vi "Test - Monitor Slip.vi"(8 "error in (no error)":errorcluster, 11 "Cluster":T1={"Preslip Sequence"=[], "Step No"=0, "Step Value"={"Sr.no"=0, "Log?"=FALSE, "Step"="", "Type"="", "Channel"="", "Value"=0.0, "Para1"=0.0, "Para2"=0.0, "Limit1"=0.0, "Limit2"=0.0, "Comparision Mode"="", "Timeout"=0.0}, "Slip Parameter"=[], "Slip Timer"=0.0, "Postslip Sequence"=[], "Postslip ?"=FALSE, "Step Result"={"Step Name"="", "Value"=0.0, "Success ?"=TRUE, "Stop Seq ?"=TRUE, "Abort"=TRUE, "Sr.No"=0}}) -> (0 "error out":errorcluster, 2 "Slip Occured ?":bool)   [LabVIEW 2017]
uses:
  Test - Message cluster.ctl
  Test - Step config.ctl
  Test - Step Result.ctl
  SubVIs/SubVI - Global.vi
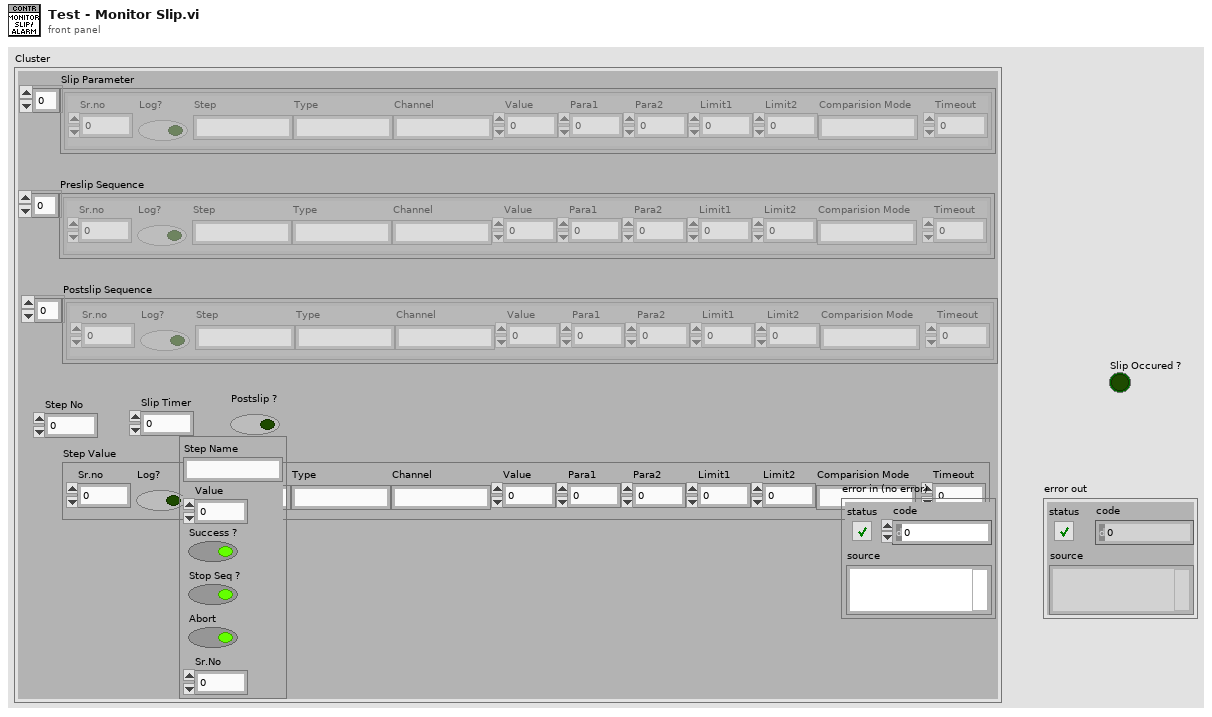
[diagram p1: front panel]
types:
  T1 = typedef "Test - Message cluster.ctl" = cluster{"Preslip Sequence":T2[], "Step No":i32, "Step Value":T2, "Slip Parameter":T2[], "Slip Timer":dbl, "Postslip Sequence":T2[], "Postslip ?":bool, "Step Result":T3}
  T2 = typedef "Test - Step config.ctl" = cluster{"Sr.no":i32, "Log?":bool, "Step":string, "Type":string, "Channel":string, "Value":dbl, "Para1":dbl, "Para2":dbl, "Limit1":dbl, "Limit2":dbl, "Comparision Mode":string, "Timeout":dbl}
  T3 = typedef "Test - Step Result.ctl" = cluster{"Step Name":string, "Value":dbl, "Success ?":bool, "Stop Seq ?":bool, "Abort":bool, "Sr.No":i32}
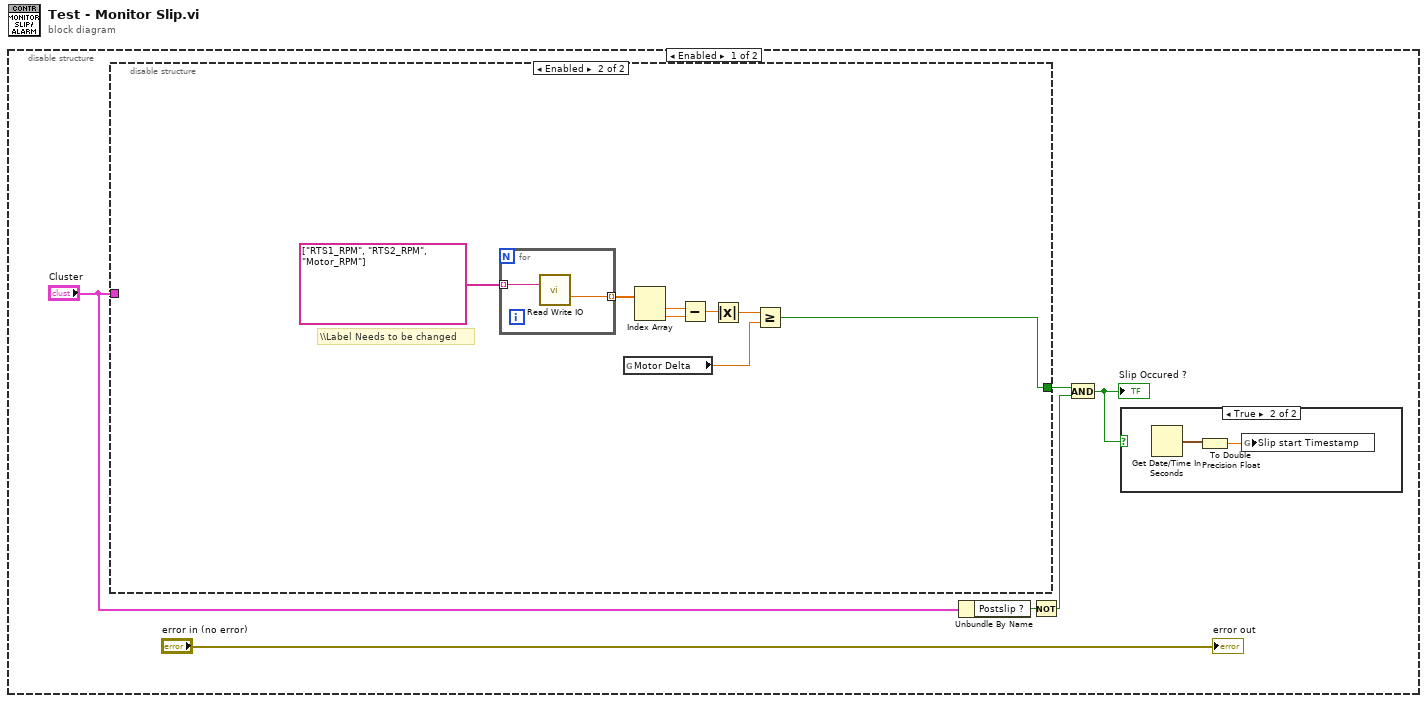
[diagram p0: block diagram]
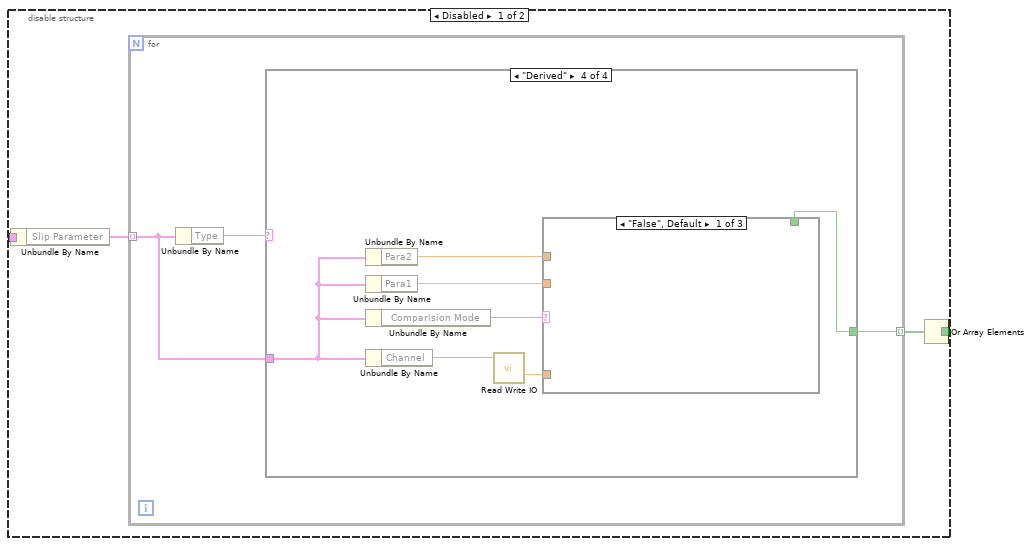
[diagram p2: hidden frame]
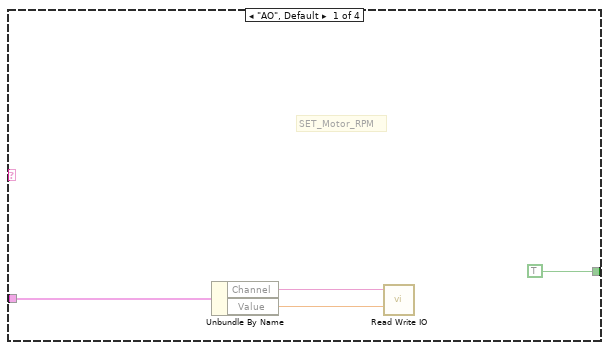
[diagram p3: hidden frame]
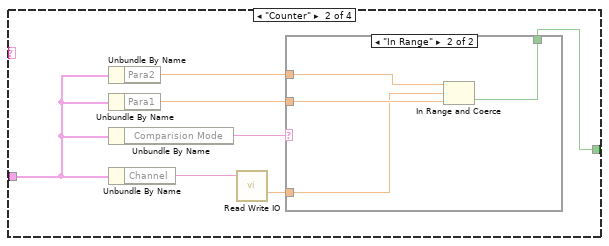
[diagram p4: hidden frame]
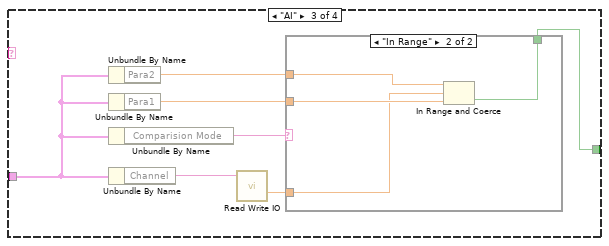
[diagram p6: hidden frame]
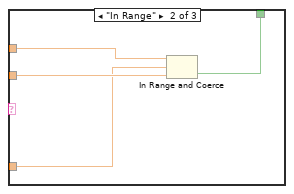
[diagram p8: hidden frame]
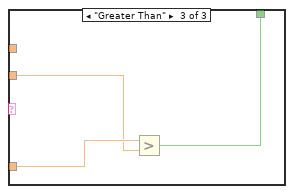
[diagram p9: hidden frame]
diagram:
  n1 = disable-structure shown="Enabled" {
    frame Enabled {
      n2 = disable-structure shown="Enabled" {
        disable-tunnel: "Cluster" -> [w8 _]
        disable-tunnel: [w7 w54] -> w2
        frame Disabled {
          n3 = Unbundle By Name(w8) -> ("Slip Parameter"=w9:T2[])
          n4 = for {
            tunnel: [w12] -> w10 mode=indexing
            tunnel: w9 -> [w11] mode=indexing
            n5 = Unbundle By Name(w11) -> ("Type"=w13:string)
            n6 = case shown="\"Derived\"" w13 {
              tunnel: w11 -> [w17 w24 w35 w46]
              tunnel: [TRUE w23 w34 w45] -> w12
              frame "AO", Default {
                # "SET_Motor_RPM"
                n7 = Unbundle By Name(w17) -> ("Channel"=w16:string, "Value"=w15:dbl)
                n8 = call "Read Write IO.vi"("Tag Name"=w16, "Value In"=w15) -> ()  [unwired: 11 in, 3 out]
              }
              frame "Counter" {
                n9 = Unbundle By Name(w24) -> ("Para2"=w19:dbl)
                n10 = Unbundle By Name(w24) -> ("Para1"=w18:dbl)
                n11 = Unbundle By Name(w24) -> ("Comparision Mode"=w21:string)
                n12 = Unbundle By Name(w24) -> ("Channel"=w22:string)
                n13 = call "Read Write IO.vi"("Tag Name"=w22) -> ("Value Out"=w20:dbl)  [unwired: 12 in, 2 out]
                n14 = case shown="\"In Range\"" w21 {
                  tunnel: w20 -> [_ w26]
                  tunnel: w19 -> [_ w28]
                  tunnel: w18 -> [_ w27]
                  tunnel: [_ w25] -> w23
                  frame "False", Default {
                  }
                  frame "In Range" {
                    n15 = In Range and Coerce(upper limit=w28, x=w26, lower limit=w27) -> (In Range?=w25:bool)  [unwired: 1 out]
                  }
                }
              }
              frame "AI" {
                n16 = Unbundle By Name(w35) -> ("Para2"=w30:dbl)
                n17 = Unbundle By Name(w35) -> ("Para1"=w29:dbl)
                n18 = Unbundle By Name(w35) -> ("Comparision Mode"=w32:string)
                n19 = Unbundle By Name(w35) -> ("Channel"=w33:string)
                n20 = call "Read Write IO.vi"("Tag Name"=w33) -> ("Value Out"=w31:dbl)  [unwired: 12 in, 2 out]
                n21 = case shown="\"In Range\"" w32 {
                  tunnel: w31 -> [_ w37]
                  tunnel: w30 -> [_ w39]
                  tunnel: w29 -> [_ w38]
                  tunnel: [_ w36] -> w34
                  frame "False", Default {
                  }
                  frame "In Range" {
                    n22 = In Range and Coerce(upper limit=w39, x=w37, lower limit=w38) -> (In Range?=w36:bool)  [unwired: 1 out]
                  }
                }
              }
              frame "Derived" {
                n23 = Unbundle By Name(w46) -> ("Para2"=w41:dbl)
                n24 = Unbundle By Name(w46) -> ("Para1"=w40:dbl)
                n25 = Unbundle By Name(w46) -> ("Comparision Mode"=w43:string)
                n26 = Unbundle By Name(w46) -> ("Channel"=w44:string)
                n27 = call "Read Write IO.vi"("Tag Name"=w44) -> ("Value Out"=w42:dbl)  [unwired: 12 in, 2 out]
                n28 = case shown="\"False\", Default" w43 {
                  tunnel: w42 -> [_ w48 w53]
                  tunnel: w41 -> [_ w50 _]
                  tunnel: w40 -> [_ w49 w52]
                  tunnel: [_ w47 w51] -> w45
                  frame "False", Default {
                  }
                  frame "In Range" {
                    n29 = In Range and Coerce(upper limit=w50, x=w48, lower limit=w49) -> (In Range?=w47:bool)  [unwired: 1 out]
                  }
                  frame "Greater Than" {
                    n30 = Greater?(x=w53, y=w52) -> (0:w51:bool)
                  }
                }
              }
            }
          }
          n31 = Or Array Elements(Boolean array=w10) -> (logical OR=w7:bool)
        }
        frame Enabled {
          # "\\\\Label Needs to be changed"
          n32 = for {
            tunnel: string[] ["RTS1_RPM", "RTS2_RPM", "Motor_RPM"] ("AI_Voltage_channels") -> [w63] mode=indexing
            tunnel: [w62] -> w60 mode=indexing
            n33 = call "Read Write IO.vi"("Tag Name"=w63) -> ("Value Out"=w62:dbl)  [unwired: 12 in, 2 out]
          }
          n34 = global read "SubVI - Global.vi" "Motor Delta"() -> (w55:dbl)
          n35 = Index Array(array=w60) -> (element #1=w59:dbl, element #2=w58:dbl)  [unwired: 2 in]
          n36 = Subtract(x=w59, y=w58) -> (x-y=w57:dbl)
          n37 = Absolute Value(x=w57) -> (abs(x)=w56:dbl)
          n38 = Greater Or Equal?(x=w56, y=w55) -> (x >= y?=w54:bool)
        }
      }
      n39 = Unbundle By Name("Cluster") -> ("Postslip ?"=w4:bool)
      n40 = Not(x=w4) -> (.not. x?=w3:bool)
      n41 = And(x=w2, y=w3) -> (x .and. y?=w1:bool)
      "Slip Occured ?" <- w1
      n42 = case shown="True" w1 {
        frame False {
        }
        frame True {
          n43 = Get Date/Time In Seconds() -> (seconds since 1Jan1904=w64:timestamp)
          n44 = To Double Precision Float(number=w64) -> (double precision float=w65:dbl)
          n45 = global write "SubVI - Global.vi" "Slip start Timestamp"(w65) -> ()
        }
      }
      "error out" <- "error in (no error)"
    }
    frame Disabled {
    }
  }
